vi "Phase Shift.vi"(6 "Axis (X)":enum16{"X", "Y"}(ring), 9 "N":i32, 11 "Graph in":cluster{dbl[], dbl[]}) -> (3 "Graph out":cluster{dbl[], dbl[]})   [LabVIEW 2015]
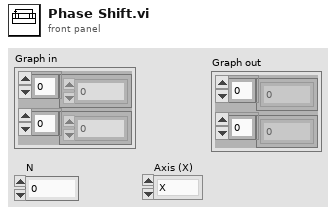
[diagram p1: front panel]
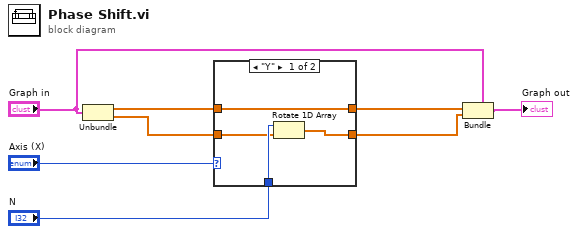
[diagram p0: block diagram]
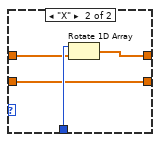
[diagram p2: hidden frame]
diagram:
  n1 = Unbundle("Graph in") -> (w7:dbl[], w6:dbl[])
  n2 = case shown="\"Y\"" "Axis (X)" {
    tunnel: "N" -> [w12 w16]
    tunnel: w7 -> [w9 w15]
    tunnel: w6 -> [w11 w13]
    tunnel: [w9 w14] -> w4
    tunnel: [w10 w13] -> w3
    frame "Y" {
      n3 = Rotate 1D Array(1:w11, 2:w12) -> (0:w10:dbl[])
    }
    frame "X" {
      n4 = Rotate 1D Array(1:w15, 2:w16) -> (0:w14:dbl[])
    }
  }
  n5 = Bundle(cluster="Graph in", w4, w3) -> (→"Graph out":cluster{dbl[], dbl[]})
